vi "Create (Group).vi"(8 "error in (no error)":errorcluster, 10 "Group Config":refnum<class "Group Config.lvclass">) -> (0 "error out":errorcluster, 3 "Scaling out":refnum<class "Scaling Config.lvclass">)   [LabVIEW 2023, in "VolatusConfig.lvlib" / "Scaling Config.lvclass"]
uses:
  Scaling Config.lvclass
  Group/Group Config.lvclass
  VolatusConfigElement/VolatusConfigElement.lvclass/VolatusConfigElement.ctl
  Scale/Scale Config.lvclass
  Scaling Config.lvclass/Scaling Config.ctl
  Channel/Channel Config.lvclass
  VolatusConfigElement/VolatusConfigElement.lvclass
  C:/dev/volatus/mts-volatus-super/libs/lv-volatus/VolatusConfig/VolatusConfigElement/VolatusConfigElement.lvclass
  C:/dev/volatus/mts-volatus-super/libs/lv-volatus/VolatusConfig/Group/Group Config.lvclass
  C:/dev/volatus/mts-volatus-super/libs/lv-volatus/VolatusConfig/Scaling/Scaling Config.lvclass
  C:/dev/volatus/mts-volatus-super/libs/lv-volatus/VolatusConfig/Channel/Channel Config.lvclass
  C:/dev/volatus/mts-volatus-super/libs/lv-volatus/VolatusConfig/Scale/Scale Config.lvclass
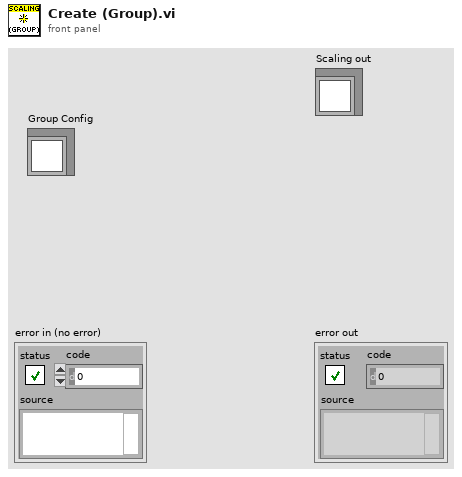
[diagram p1: front panel]
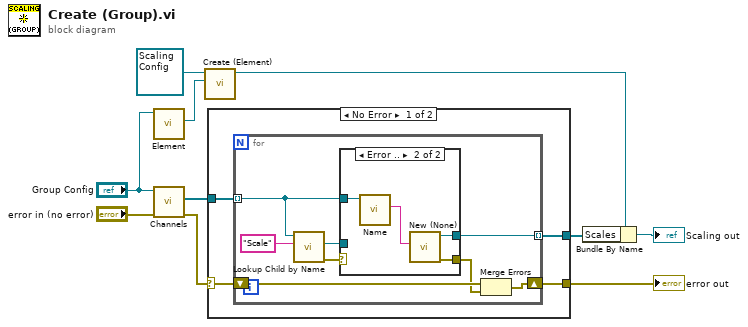
[diagram p0: block diagram]
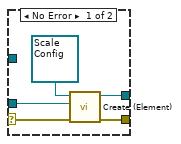
[diagram p2: hidden frame]
diagram:
  n1 = call "Element.vi"("VolatusConfigElement in"="Group Config") -> ("Element"=w6:refnum<class "Config Element.lvclass">)  [unwired: 9 in, 1 out]
  n2 = call "Channels.vi"("error in (no error)"="error in (no error)", "Group in"="Group Config") -> ("error out"=w10:errorcluster, "Channels"=w9:refnum<class "Channel Config.lvclass">[])  [unwired: 7 in, 1 out]
  n3 = call "Create (Element).vi"("Element"=w6, "VolatusConfigElement in"=refnum<class "Scaling Config.lvclass"> refnum ("Scaling in")) -> ("VolatusConfigElement out"=w4:refnum<class "Scaling Config.lvclass">)  [unwired: 8 in, 1 out]
  n4 = case shown="No Error" w10 {
    selector: w10 -> [w14 w32]
    tunnel: w9 -> [w13 _]
    tunnel: [w12 _] -> w5
    tunnel: [w11 w32] -> w1
    frame No Error {
      n5 = for {
        shift-right: [w15] -> w11
        shift-left: w14 -> [w17]
        tunnel: w13 -> [w18] mode=indexing
        tunnel: [w21] -> w12 mode=indexing
        n6 = call "Lookup Child by Name.vi"("Child Name"="Scale", "VolatusConfigElement in"=w18) -> ("error out"=w20:errorcluster, "Child"=w22:refnum<class "Config Element.lvclass">)  [unwired: 6 in, 2 out]
        n7 = case shown="Error .." w20 {
          selector: w20 -> [w25 _]
          tunnel: w22 -> [w27 _]
          tunnel: [w26 w30] -> w21
          tunnel: w18 -> [_ w29]
          tunnel: [w23 w31] -> w16
          frame No Error {
            n8 = call "Create (Element).vi"("error in (no error)"=w25, "Element"=w27, "VolatusConfigElement in"=refnum<class "Scale Config.lvclass"> refnum ("VolatusConfig.lvlib:Scale.lvclass")) -> ("error out"=w23:errorcluster, "VolatusConfigElement out"=w26:refnum<class "Scale Config.lvclass">)  [unwired: 7 in]
          }
          frame Error {
            n9 = call "Name.vi"("VolatusConfigElement in"=w29) -> ("Name"=w28:string)  [unwired: 8 in, 2 out]
            n10 = call "New (None).vi"("Channel Name"=w28) -> ("error out"=w31:errorcluster, "Scale out"=w30:refnum<class "Scale Config.lvclass">)  [unwired: 9 in]
          }
        }
        n11 = Merge Errors(w17, w16) -> (w15:errorcluster)
      }
    }
    frame Error {
    }
  }
  "error out" <- w1
  n12 = Bundle By Name(cluster=w4, "Scales"=w5) -> (→"Scaling out":refnum<class "Scaling Config.lvclass">)
